vi "校准数据选择表.vi"(9 "测量模式":T1(ring), 10 "量程下拉列表":enum16{"低量程", "高量程"}(ring), 11 "table":string="氨氮") -> (2 "布尔":bool=TRUE, 3 "输出":T2)   [LabVIEW 2016, in "斯坦道通用流路CODmn.lvlib"]
uses:
  <vilib>/Utility/miscctls.llb/LVPointTypeDef.ctl
  <vilib>/Utility/miscctls.llb/LVRowAndColumnUnsignedTypeDef.ctl
panel:
  in  "显示所有数据":bool caption="显示所有数据："
  in  "确定":bool
  in  "返回":bool
  in  "多列列表框":i32(listbox)
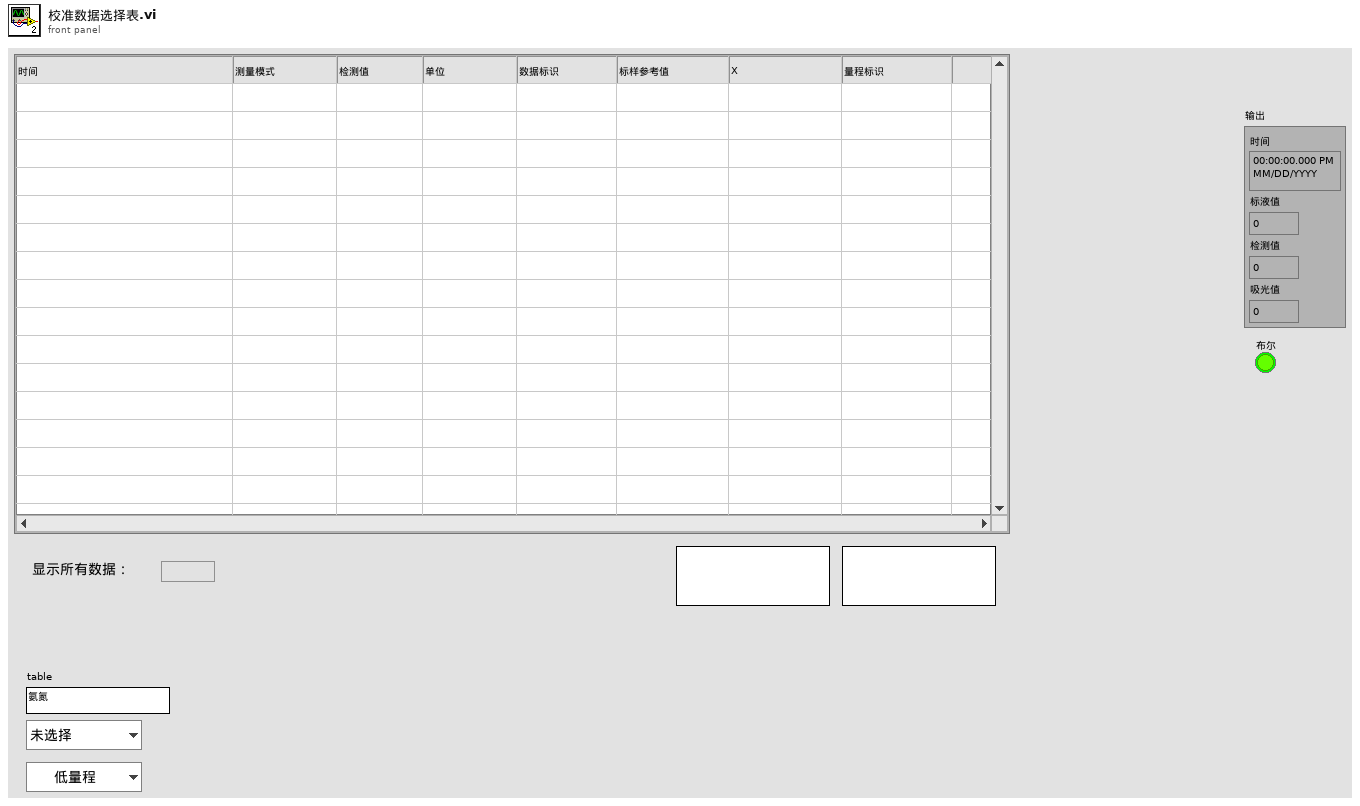
[diagram p1: front panel]
types:
  T1 = enum16{"未选择", "空白校准", "标样校准", "标样核查", "零点核查", "跨度核查"}
  T2 = cluster{"时间":timestamp, "标液值":dbl, "检测值":dbl, "吸光值":dbl}
  T3 = typedef "LVRowAndColumnUnsignedTypeDef.ctl" = cluster{"Row":u32, "Column":u32}
  T4 = typedef "LVPointTypeDef.ctl" = cluster{"Horizontal":i16, "Vertical":i16}
  T5 = typedef "SingleStepTestV3.lvlib/SingleStepTestV3.lvclass/仪器版本.ctl" = enum16{"V3.1版", "V4版", "V3版", "V4.2版"}
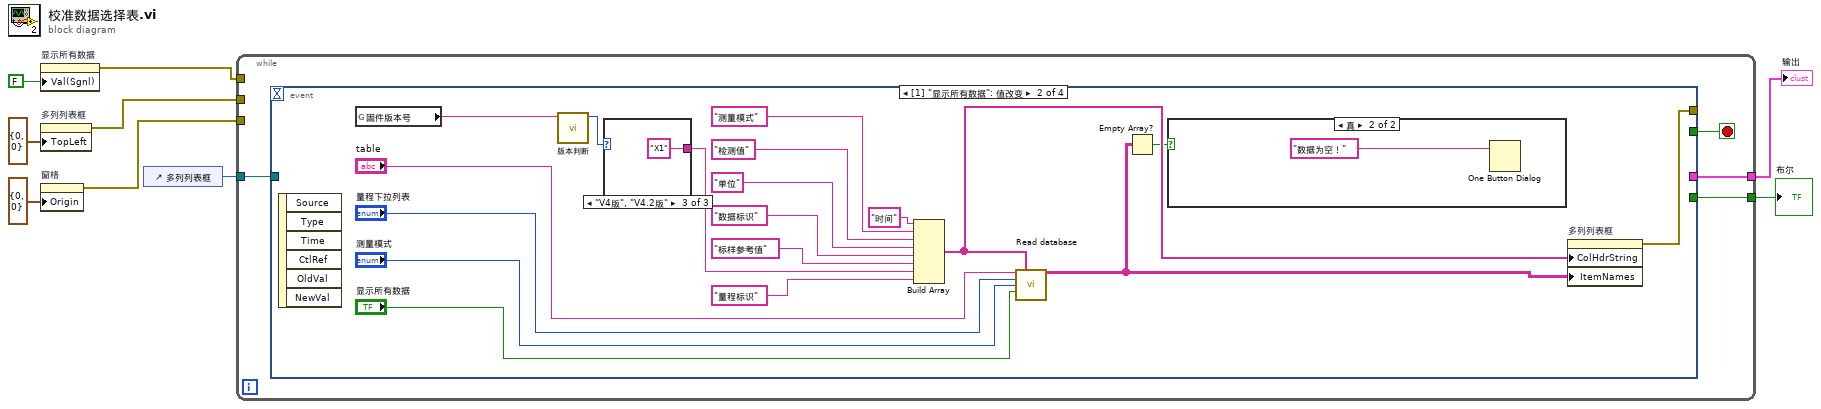
[diagram p0: block diagram]
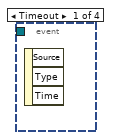
[diagram p2: hidden frame]
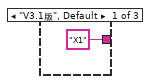
[diagram p3: hidden frame]
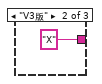
[diagram p4: hidden frame]
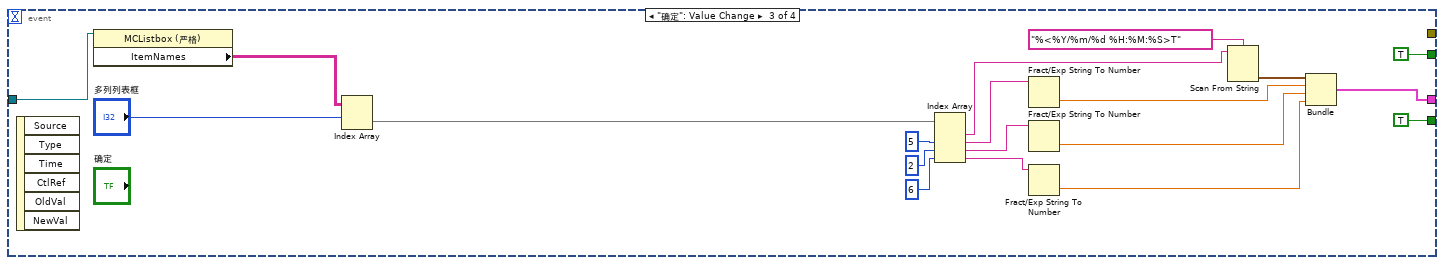
[diagram p6: hidden frame]
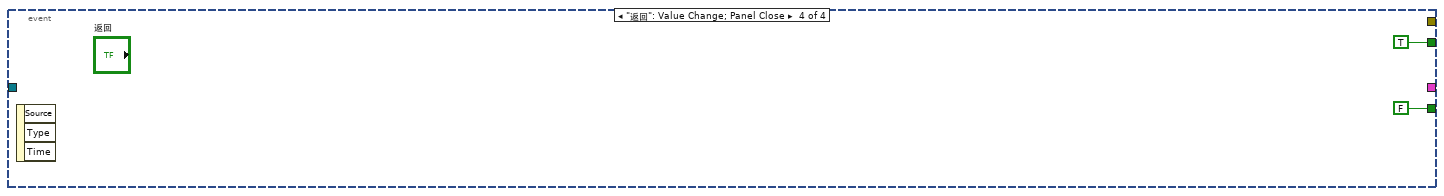
[diagram p7: hidden frame]
diagram:
  n1 = property on="显示所有数据" class="Bool (严格)"("Val(Sgnl)"=FALSE ("值(信号)")) -> (error out=w1:errorcluster)  [unwired: 2 in, 1 out]
  n2 = property on="多列列表框" class="MCListbox (严格)"("TopLeft"=T3 {"Row"=0, "Column"=0} ("左上可见单元格")) -> (error out=w3:errorcluster)  [unwired: 2 in, 1 out]
  n3 = property on="窗格" class="Pane"("Origin"=T4 {"Horizontal"=0, "Vertical"=0} ("原点")) -> (error out=w8:errorcluster)  [unwired: 2 in, 1 out]
  n4 = control-ref of="多列列表框"() -> (w5:refnum<vi>)
  n5 = while {
    tunnel: w5 -> [w12]
    tunnel: w8 -> [_]
    tunnel: [w11] -> w7
    tunnel: [w10] -> w6
    tunnel: w3 -> [_]
    tunnel: w1 -> [_]
    stop <- w13 stop-if-true
    n6 = event shown="[1] \"显示所有数据\": 值改变" {
      selector: _ -> [_ _ _ _]
      dyn-events: _ -> [_ _ _ _]
      timeout: _ -> [_ _ _ _]
      tunnel: [_ _ TRUE TRUE] -> w13
      tunnel: w12 -> [_ _ w52 _]
      tunnel: [_ _ TRUE FALSE] -> w11
      tunnel: [_ _ w39 _] -> w10
      tunnel: [_ w17 _ _] -> _
      event Timeout {
        n7 = event-data() -> ()  [unwired: 1 in, 3 out]
      }
      event "显示所有数据": Value Change {
        n8 = event-data() -> ()  [unwired: 1 in, 6 out]
        n9 = global read "VAR总磷总氮全局变量.vi" "固件版本号"() -> (w16:string)
        n10 = call "版本判断.vi"("固件版本号"=w16) -> ("仪器版本"=w15:T5)  [unwired: 10 in]
        n11 = case shown="\"V4版\", \"V4.2版\"" w15 {
          tunnel: ["X1" "X" "X1"] -> w14
          frame "V3.1版", Default {
          }
          frame "V3版" {
          }
          frame "V4版", "V4.2版" {
          }
        }
        n12 = Build Array("时间", "测量模式", "检测值", "单位", "数据标识", "标样参考值", w14, "量程标识") -> (w26:string[])
        n13 = call "Read database.vi"("table"="table", "显示项"=w26, "量程下拉列表"="量程下拉列表", "测量模式"="测量模式", "显示所有数据"="显示所有数据") -> ("表格"=w18:string[][])  [unwired: 7 in, 3 out]
        n14 = Empty Array?(array=w18) -> (empty?=w19:bool)
        n15 = case shown="真" w19 {
          frame False {
          }
          frame True {
            n16 = One Button Dialog(message="数据为空！" ("消息")) -> ()  [unwired: 1 in, 1 out]
          }
        }
        n17 = property on="多列列表框" class="MCListbox (严格)"("ColHdrString"=w26, "ItemNames"=w18) -> (error out=w17:errorcluster)  [unwired: 2 in, 1 out]
      }
      event "确定": Value Change {
        n18 = event-data() -> ()  [unwired: 1 in, 6 out]
        n19 = property class="MCListbox (严格)"(reference=w52) -> ("ItemNames"=w53:string[][])  [unwired: 1 in, 2 out]
        n20 = Index Array(array=w53, index (row)="多列列表框") -> (element=w49:string[])  [unwired: 1 in]
        n21 = Index Array(array=w49, index #2=5 ("索引"), index #3=2 ("索引"), index #4=6 ("索引")) -> (element #1=w37:string, element #2=w45:string, element #3=w44:string, element #4=w43:string)  [unwired: 1 in]
        n22 = Fract/Exp String To Number(string=w45) -> (number=w42:dbl)  [unwired: 3 in, 1 out]
        n23 = Fract/Exp String To Number(string=w44) -> (number=w41:dbl)  [unwired: 3 in, 1 out]
        n24 = Fract/Exp String To Number(string=w43) -> (number=w40:dbl)  [unwired: 3 in, 1 out]
        n25 = Scan From String(format string="%<%Y/%m/%d %H:%M:%S>T" ("格式字符串"), input string=w37) -> (output 1=w36:timestamp)  [unwired: 3 in, 3 out]
        n26 = Bundle(w36, w42, w41, w40) -> (w39:cluster{timestamp, dbl, dbl, dbl})  [unwired: 1 in]
      }
      event "返回": Value Change; Panel Close {
        n27 = event-data() -> ()  [unwired: 1 in, 3 out]
      }
    }
  }
  "布尔" <- w7
  "输出" <- w6
